vi "System Properties UI.vi"(8 "error in (no error)":errorcluster, 11 "Editor Handler in":refnum<class "Imager Handler.lvclass">=refnum) -> (0 "error out":errorcluster, 3 "Editor Handler out":refnum<class "Imager Handler.lvclass">)   [LabVIEW 2016, in "Imager Handler.lvclass"]
uses:
  Imager Handler.lvclass
  C:/Program Files (x86)/National Instruments/LabVIEW 2016/vi.lib/LIEF/Image Editor Handler/Image Editor Handler.lvclass
  <vilib>/LIEF/Image/Image.lvclass
  <vilib>/LIEF/Image Editor Handler/Image Editor Handler.lvclass/Image Editor Handler.ctl
  Imager Handler.lvclass/Imager Handler.ctl
  <vilib>/LIEF/Image Editor Handler/Read Events.vi
  <vilib>/LIEF/Forms/Shape/Shape.lvclass
panel:
  out "Name":string
  out "Address":string
  in  "Properties Table":i32[](listbox)
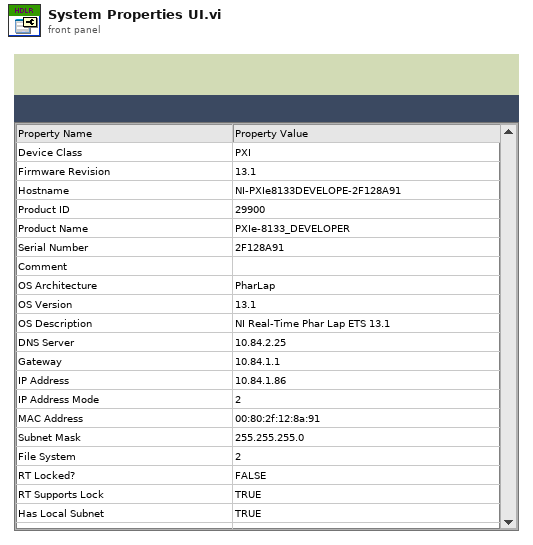
[diagram p1: front panel]
types:
  T1 = typedef "LV Image Editor Framework.lvlib/Image Editor Handler.lvclass/Editor Events.ctl" = cluster{"Stop":refnum<user-event>, "Image Events":cluster{"AddShape":refnum<user-event>, "Paint":refnum<user-event>, "RemoveShape":refnum<user-event>, "RefreshShape ByRef":refnum<user-event>, "ShapePropertyChange":refnum<user-event>, "RemoveShape ByRef":refnum<user-event>}, "RequestShapes":refnum<user-event>, "Custom":refnum<user-event>}
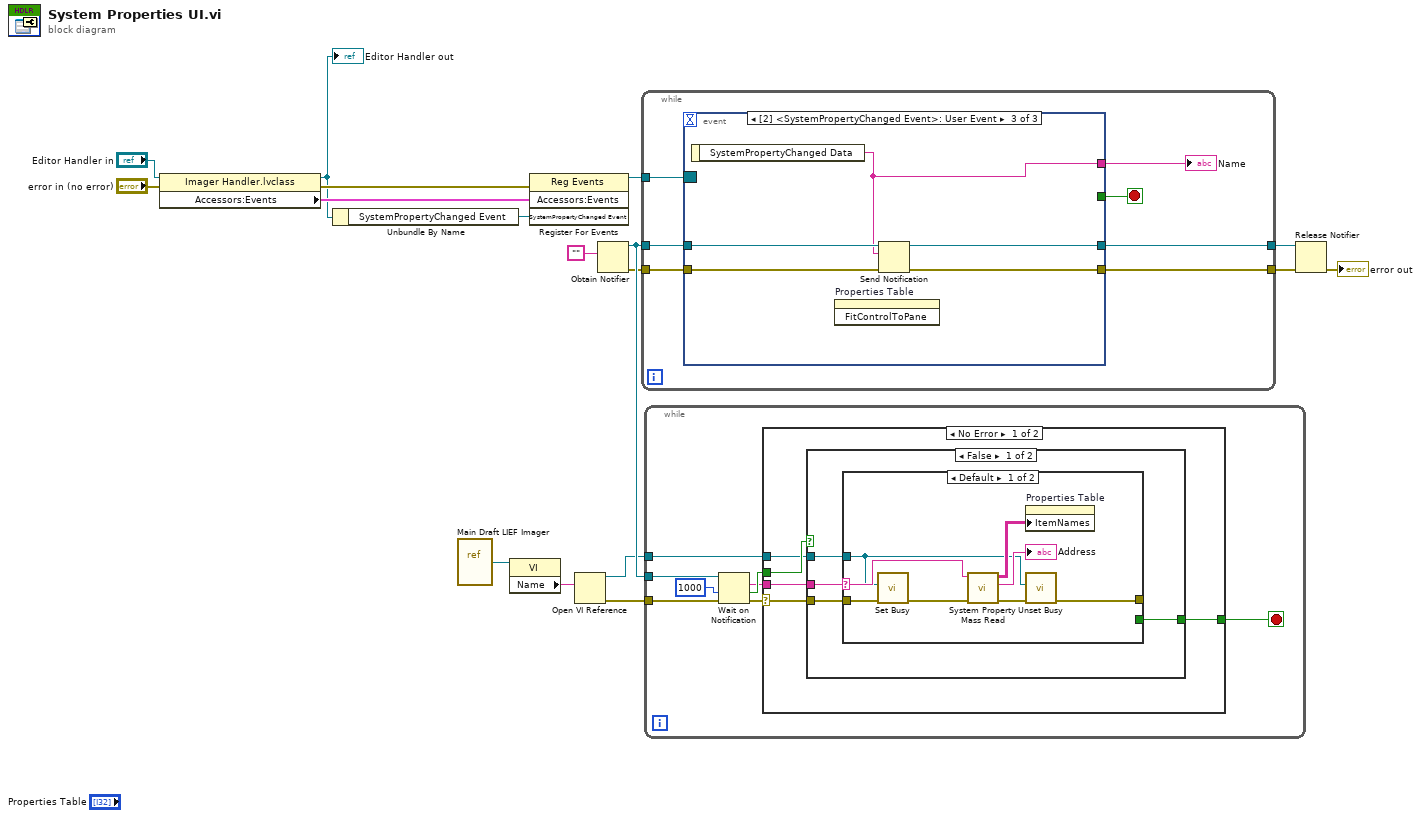
[diagram p0: block diagram]
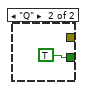
[diagram p2: hidden frame]
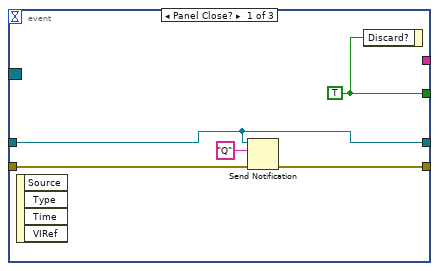
[diagram p5: hidden frame]
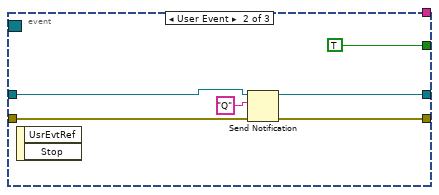
[diagram p6: hidden frame]
diagram:
  n1 = property class="Imager Handler.lvclass"(reference="Editor Handler in", error in="error in (no error)") -> (reference out=w1:refnum<class "Imager Handler.lvclass">, error out=w14:errorcluster, "Accessors:Events"=w16:T1)
  "Editor Handler out" <- w1
  n2 = Unbundle By Name(w1) -> ("SystemPropertyChanged Event"=w12:refnum<user-event>)
  n3 = vi-ref "Main Draft LIEF Imager.vi"() -> (w8:refnum<vi>)
  n4 = property class="VI"(reference=w8) -> ("Name"=w7:string)  [unwired: 1 in, 2 out]
  n5 = register-events(error in=w14, w16, w12) -> (reference out=w15:refnum<event-registration>)  [unwired: 1 in, 1 out]
  n6 = Open VI Reference(vi path=w7) -> (vi reference=w6:refnum<vi>, error out=w5:errorcluster)  [unwired: 5 in]
  n7 = Obtain Notifier(notification data type="") -> (notifier out=w10:refnum<notifier>, error out=w4:errorcluster)  [unwired: 3 in, 1 out]
  n8 = while {
    tunnel: w15 -> [w24]
    tunnel: w10 -> [w21]
    tunnel: [w20] -> w9
    tunnel: w4 -> [w19]
    tunnel: [w18] -> w3
    stop <- w23 stop-if-true
    n9 = event shown="[2] <SystemPropertyChanged Event>: User Event" {
      selector: w24 -> [_ _ _]
      dyn-events: _ -> [_ _ _]
      timeout: _ -> [_ _ _]
      tunnel: [w29 TRUE ("Discard?") _] -> w23
      tunnel: [_ _ w39] -> w22
      tunnel: w21 -> [w28 w33 w40]
      tunnel: [w28 w32 w38] -> w20
      tunnel: w19 -> [w26 w31 w37]
      tunnel: [w25 w30 w36] -> w18
      event Panel Close? {
        w29 = TRUE ("Discard?")
        n10 = event-data() -> ()  [unwired: 1 in, 4 out]
        n11 = Send Notification(notification="Q", notifier=w28, error in (no error)=w26) -> (error out=w25:errorcluster)  [unwired: 1 out]
        n12 = event-data("Discard?"=w29) -> ()  [unwired: 1 in, 1 out]
      }
      event User Event {
        n13 = event-data() -> ()  [unwired: 1 in, 2 out]
        n14 = Send Notification(notification="Q", notifier=w33, error in (no error)=w31) -> (notifier out=w32:refnum<notifier>, error out=w30:errorcluster)
      }
      event User Event {
        n15 = event-data() -> ("SystemPropertyChanged Data"=w39:string)  [unwired: 1 in]
        n16 = invoke on="Properties Table" class="MCListbox (strict)" method="FitControlToPane"() -> ()  [unwired: 3 in, 3 out]
        n17 = Send Notification(notification=w39, notifier=w40, error in (no error)=w37) -> (notifier out=w38:refnum<notifier>, error out=w36:errorcluster)
      }
    }
    "Name" <- w22
  }
  n18 = while {
    tunnel: w10 -> [w48]
    tunnel: w6 -> [w42]
    tunnel: w5 -> [w41]
    stop <- w44 stop-if-true
    n19 = Wait on Notification(notifier=w48, timeout in ms (-1)=1000, error in (no error)=w41) -> (notification=w45:string, timed out?=w46:bool, error out=w47:errorcluster)  [unwired: 1 in, 1 out]
    n20 = case shown="No Error" w47 {
      selector: w47 -> [w50 _]
      tunnel: w46 -> [w53 _]
      tunnel: w45 -> [w52 _]
      tunnel: [w51 _] -> w44
      tunnel: w42 -> [w49 _]
      frame No Error {
        n21 = case shown="False" w53 {
          tunnel: w52 -> [w57 _]
          tunnel: [w56 _] -> w51
          tunnel: w50 -> [w55 _]
          tunnel: w49 -> [w54 _]
          frame False {
            n22 = case shown="Default" w57 {
              selector: w57 -> [w65 _]
              tunnel: [_ TRUE] -> w56
              tunnel: w55 -> [w62 _]
              tunnel: w54 -> [w60 _]
              tunnel: [w58 _] -> _
              frame Default {
                n23 = call <vilib>:"Set Busy.vi"("error in (no error)"=w62, "VI reference (current VI)"=w60) -> ("error out"=w59:errorcluster)  [unwired: 8 in, 1 out]
                n24 = call "System Property Mass Read.vi"("error in (no error)"=w59, "System Name"=w65) -> ("error out"=w61:errorcluster, "IP Address"=→"Address":string, "Properties Pairs"=w64:string[][])  [unwired: 7 in]
                n25 = property on="Properties Table" class="MCListbox (strict)"("ItemNames"=w64) -> ()  [unwired: 2 in, 2 out]
                n26 = call <vilib>:"Unset Busy.vi"("error in (no error)"=w61, "VI reference (current VI)"=w60) -> ("error out"=w58:errorcluster)  [unwired: 9 in]
              }
              frame "Q" {
              }
            }
          }
          frame True {
          }
        }
      }
      frame Error {
      }
    }
  }
  n27 = Release Notifier(notifier=w9, error in (no error)=w3) -> (error out=→"error out":errorcluster)  [unwired: 1 in, 2 out]
